vi "TankDriveHandler.vi"(6 "Sensitivity (.01)":dbl=0.01, 7 "TankDrive Queue":refnum<queue>, 8 "Error In (no error)":errorcluster, 9 "Right Motor Value":dbl, 10 "Left Motor Value":dbl, 11 "HalfSpeed (F)":bool) -> (0 "Error Out":errorcluster)   [LabVIEW 2012]
doc: "Handles input for tank drive. \nParameters:\n- Motor values: default to 0 if unwired.\n- Mode: Init or Do. Init will set the motors to 0 and prepare this VI for future calls, so this VI should be called with Init first. Do will update the motor values according to LeftMotorValue and RightMotorValue.\n- HalfSpeed: If true, cuts motor speed in half. Defaults to false.\n- Sensitivity: A measure of how big a change in joystick value is needed to trigger an event. Defaults to .01.\n-TankDrive Queue: the queue on which instructions will be enqueued\nIf the motor values changed significantly, a tank drive enstruction will be enqueued."
uses:
  QueueInstruction.ctl
  SubsystemEnum.ctl
  ActionEnum.ctl
  TankDriveInstruction.ctl
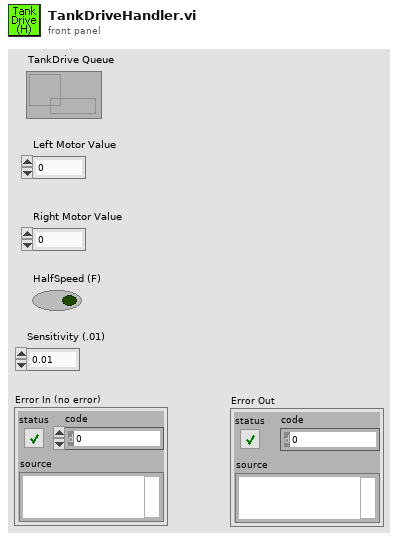
[diagram p1: front panel]
types:
  T1 = typedef "ActionEnum.ctl" = enum16{"Init", "SetValue"}
  T2 = typedef "SubsystemEnum.ctl" = enum16{"TankDrive", "FirePneumatic", "Climber", "ClimbWeight", "ShooterAngle"}
  T3 = typedef "TankDriveInstruction.ctl" = cluster{"LeftMotorValue":dbl, "RightMotorValue":dbl, "HalfSpeed":bool}
  T4 = typedef "QueueInstruction.ctl" = cluster{"Data":variant, "Subsystem":T2, "Action":T1}
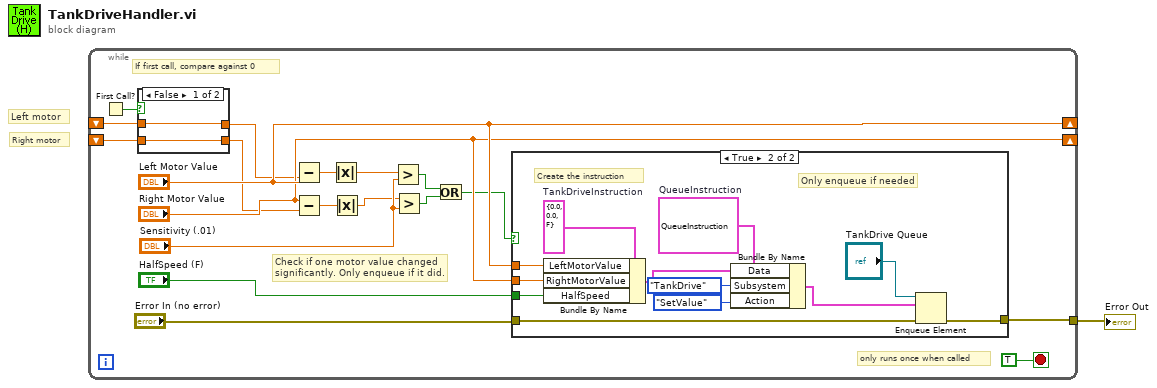
[diagram p0: block diagram]
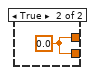
[diagram p3: hidden frame]
diagram:
  # "Right motor"
  # "Left motor"
  n1 = while {
    shift-right: ["Left Motor Value"] -> _
    shift-left: _ -> [w7]
    shift-right: ["Right Motor Value"] -> _
    shift-left: _ -> [w5]
    tunnel: [w15] -> w1
    stop <- TRUE stop-if-true
    # "If first call, compare against 0"
    # "Check if one motor value changed\nsignificantly. Only enqueue if it did."
    # "only runs once when called"
    n2 = First Call?() -> (First Call?: T/F=w3:bool)
    n3 = case shown="False" w3 {
      tunnel: w7 -> [w35 _]
      tunnel: [w35 w36] -> w6
      tunnel: w5 -> [w34 _]
      tunnel: [w34 w36] -> w4
      frame False {
      }
      frame True {
        w36 = 0.0
      }
    }
    n4 = Subtract(x="Left Motor Value", y=w6) -> (x-y=w13:dbl)
    n5 = Subtract(x="Right Motor Value", y=w4) -> (x-y=w12:dbl)
    n6 = Absolute Value(x=w13) -> (abs(x)=w11:dbl)
    n7 = Absolute Value(x=w12) -> (abs(x)=w10:dbl)
    n8 = Greater?(x=w11, y="Sensitivity (.01)") -> (0:w8:bool)
    n9 = Greater?(x=w10, y="Sensitivity (.01)") -> (0:w9:bool)
    n10 = Or(x=w8, y=w9) -> (x .or. y?=w2:bool)
    n11 = case shown="True" w2 {
      tunnel: "Error In (no error)" -> [w21 w33]
      tunnel: "Left Motor Value" -> [_ w32]
      tunnel: "Right Motor Value" -> [_ w31]
      tunnel: [w21 w30] -> w15
      tunnel: "HalfSpeed (F)" -> [_ w29]
      frame False {
      }
      frame True {
        w28 = T3 {"LeftMotorValue"=0.0, "RightMotorValue"=0.0, "HalfSpeed"=FALSE}  # TankDriveInstruction
        w27 = T4 {"Data"=variant, "Subsystem"=enum."TankDrive", "Action"=enum."Init"}  # QueueInstruction
        # "Only enqueue if needed"
        # "Create the instruction"
        n12 = Bundle By Name(cluster=w28, "LeftMotorValue"=w32, "RightMotorValue"=w31, "HalfSpeed"=w29) -> (w26:T3)
        n13 = Bundle By Name(cluster=w27, "Data"=w26, "Subsystem"=SubsystemEnum."TankDrive", "Action"=ActionEnum."SetValue") -> (w23:T4)
        n14 = Enqueue Element(queue="TankDrive Queue", element=w23, error in (no error)=w33) -> (error out=w30:errorcluster)  [unwired: 1 in, 2 out]
      }
    }
  }
  "Error Out" <- w1
